vi "Read channel array.vi"(8 "error in (no error)":errorcluster, 11 "Y (Complex) (N Ch) in":refnum<class "Y (Complex) (N Ch).lvclass">) -> (0 "error out":errorcluster, 2 "channel array":T1(array[cluster]), 3 "Y (Complex) (N Ch) out":refnum<class "Y (Complex) (N Ch).lvclass">)   [LabVIEW 2017, in "Y (Complex) (N Ch).lvclass"]
uses:
  <vilib>/addons/_NISVFA/_Shared subVIs/Data Objects/Y (Complex) (DBL)/Y (Complex) (N Ch).lvclass
  <vilib>/addons/_NISVFA/_Shared subVIs/Data Objects/Y (Complex) (DBL)/Y (Complex) (N Ch).lvclass/Y (Complex) (N Ch).ctl
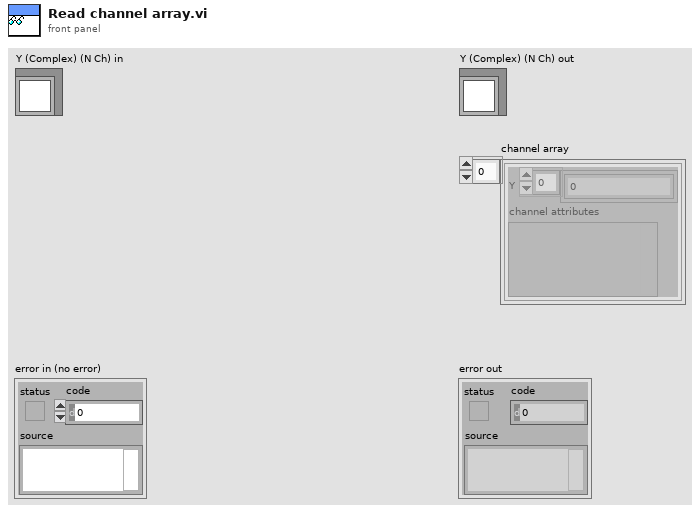
[diagram p1: front panel]
types:
  T1 = cluster{"Y":cdb[], "channel attributes":variant}[]
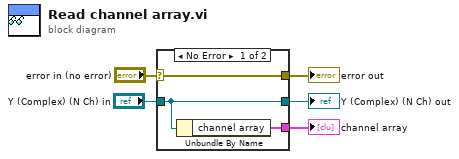
[diagram p0: block diagram]
diagram:
  n1 = case shown="No Error" "error in (no error)" {
    selector: "error in (no error)" -> [w8 w9]
    tunnel: [w8 w9] -> w4
    tunnel: [w7 w10] -> w2
    tunnel: "Y (Complex) (N Ch) in" -> [w7 w10]
    tunnel: [w6 _] -> w1
    frame No Error {
      n2 = Unbundle By Name(w7) -> ("channel array"=w6:T1)
    }
    frame Error {
    }
  }
  "error out" <- w4
  "Y (Complex) (N Ch) out" <- w2
  "channel array" <- w1
